vi "Wait Action.vi"() -> (3 "Run Result":T1)   [LabVIEW 2020, in "SquareBattle.lvlib"]
doc: "Utility method to easily create a wait action run result. When a square is waiting, it remains in place until the next round. A waiting square can still be attacked or collided with."
uses:
  SquareBattle.lvlib
  Run Result.ctl
  Square/Square.lvclass
  Action.ctl
  Direction.ctl
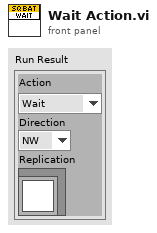
[diagram p1: front panel]
types:
  T1 = typedef "SquareBattle.lvlib/Run Result.ctl" = cluster{"Action":T2, "Direction":T3, "Replication":refnum<class "Square.lvclass">}
  T2 = typedef "SquareBattle.lvlib/Action.ctl" = enum16{"Wait", "Move", "Attack", "Replicate"}
  T3 = typedef "SquareBattle.lvlib/Direction.ctl" = enum16{"NW", "N", "NE", "E", "SE", "S", "SW", "W"}
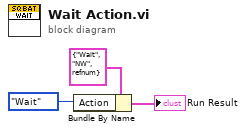
[diagram p0: block diagram]
diagram:
  n1 = Bundle By Name(cluster=T1 {"Action"=enum."Wait", "Direction"=enum."NW", "Replication"=refnum} ("Run Result"), "Action"=Action."Wait") -> (→"Run Result":T1)
